vi "4461 - Create AO DC waveforms.vi"(8 "error in (no error)":errorcluster, 9 "sweep index":i32=-1, 10 "reset signal":bool, 11 "LockinDAQ":refnum<class "LockinDAQ.lvclass">) -> (0 "error out":errorcluster, 2 "AO Array":waveform(dbl)[](array[waveform]), 3 "LockinDAQ out":refnum<class "LockinDAQ.lvclass">)   [LabVIEW 2016, in "LockinDAQ.lvclass"]
uses:
  LockinDAQ.lvclass
  LockinDAQ.lvclass/LockinDAQ.ctl
  <vilib>/Analysis/1siggen.llb/Ramp Pattern by Samples.vi
  <vilib>/Analysis/NI_AALBase.lvlib
  <vilib>/measure/NI_MABase.lvlib
panel:
  in  "Update graphs?":bool
  out "Waveform Graph":waveform(dbl)[](graph)
  out "Numeric":i32
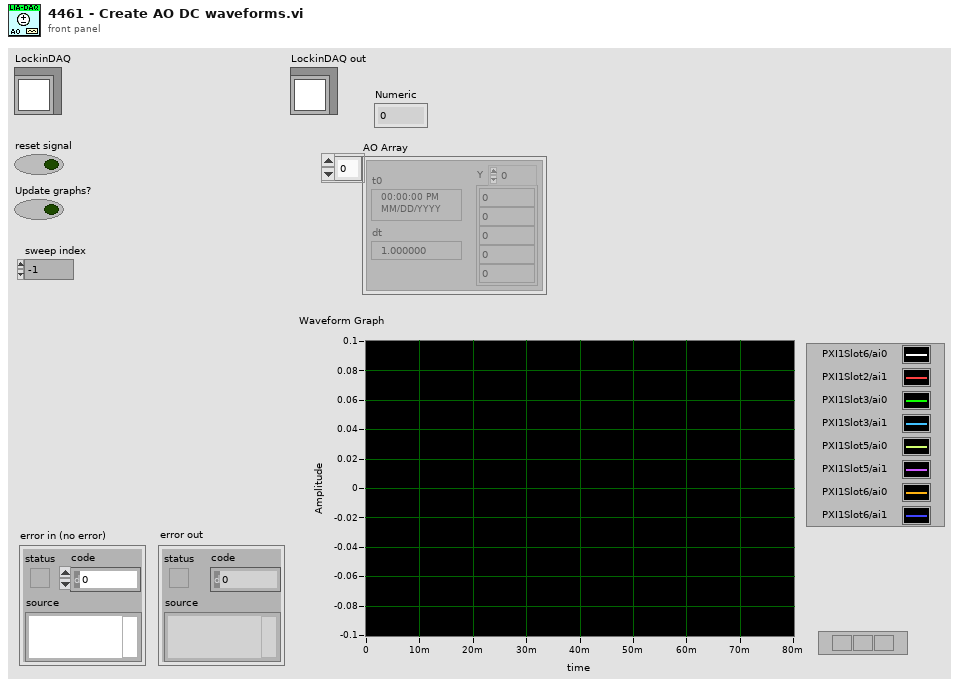
[diagram p1: front panel]
types:
  T1 = typedef "LockinDAQ.lvclass/Sampling.ctl" = cluster{"Fs":dbl, "#s":i32}
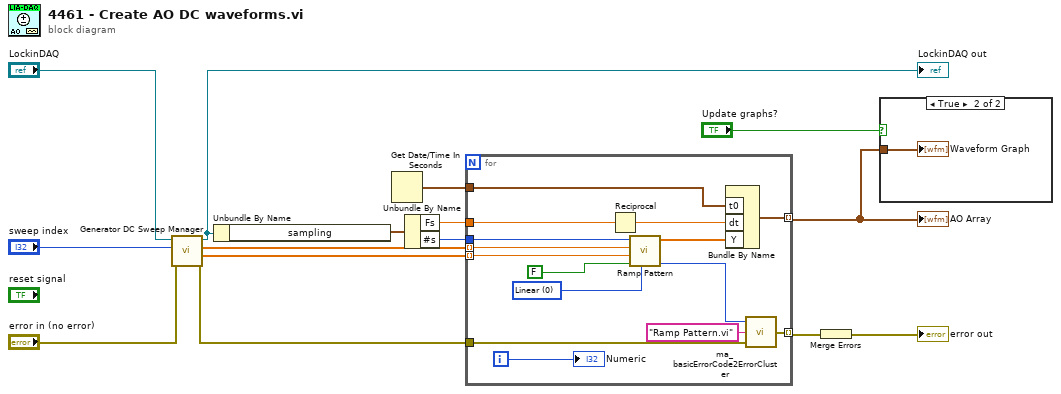
[diagram p0: block diagram]
diagram:
  n1 = call "Generator DC Sweep Manager.vi"("error in (no error)"="error in (no error)", "sweep index"="sweep index", "LockinDAQ"="LockinDAQ") -> ("error out"=w4:errorcluster, "Start (V)"=w7:dbl[], "End (V)"=w3:dbl[], "LockinDAQ out"=w1:refnum<class "LockinDAQ.lvclass">)  [unwired: 5 in]
  "LockinDAQ out" <- w1
  n2 = Unbundle By Name(w1) -> ("sampling"=w9:T1)
  n3 = Get Date/Time In Seconds() -> (seconds since 1Jan1904=w11:timestamp)
  n4 = Unbundle By Name(w9) -> ("Fs"=w6:dbl, "#s"=w5:i32)
  n5 = for {
    tunnel: [w29] -> w13 mode=indexing
    tunnel: w4 -> [w26]
    tunnel: [w24] -> w8 mode=indexing
    tunnel: w11 -> [w16]
    tunnel: w3 -> [w20] mode=indexing
    tunnel: w7 -> [w19] mode=indexing
    tunnel: w6 -> [w18]
    tunnel: w5 -> [w17]
    i -> [w30]
    w22 = u16 0 items=["Linear", "Logarithmic"] ("type")
    n6 = Reciprocal(x=w18) -> (1/x=w25:dbl)
    n7 = call-poly <vilib>:"Ramp Pattern.vi"("type"=w22, "exclude end?"=FALSE, "start"=w19, "end"=w20, "samples"=w17) -> ("error"=w23:i32, "Ramp Pattern"=w28:dbl[])  [unwired: 5 in]
    n8 = Bundle By Name("t0"=w16, "dt"=w25, "Y"=w28) -> (w29:waveform(dbl))  [unwired: 1 in]
    n9 = call <vilib>:"ma_basicErrorCode2ErrorCluster.vi"("error in (no error)"=w26, "subVI name"="Ramp Pattern.vi", "Error Code"=w23) -> ("error out"=w24:errorcluster)
    "Numeric" <- w30
  }
  "AO Array" <- w13
  n10 = Merge Errors(w8) -> (→"error out":errorcluster)
  n11 = case shown="True" "Update graphs?" {
    tunnel: w13 -> [_ w31]
    frame False {
    }
    frame True {
      "Waveform Graph" <- w31
    }
  }
